vi "Test Real Matrix Type.vi"(9 "relative tolerance":dbl=-1.0, 10 "matrix type":T1=10 items=["Symmetric Positive Definite"=10, "Symmetric Positive Semi-Definite"=11, "Symmetric"=20, "Hermitian"=21], 11 "Input Matrix":T2) -> (0 "error":i32, 3 "is type?":bool)   [LabVIEW 2017, in "NI_AALPro.lvlib"]
doc: "Tests whether<B> Input Matrix</B> is a matrix of special type. Wire data to the <B>Input Matrix</B> input to determine the polymorphic instance to use or manually select the instance."
uses:
  NI_AALPro.lvlib
  RealMatrix.ctl
  Matrix Type for Test.ctl
  NI_Matrix.lvlib
panel:
  # "Test Matrix Type"
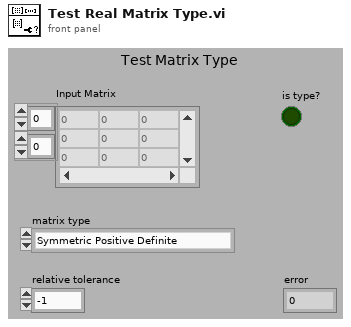
[diagram p1: front panel]
types:
  T1 = typedef "NI_AALPro.lvlib/Matrix Type for Test.ctl" = i32
  T2 = typedef "NI_Matrix.lvlib/RealMatrix.ctl" = dbl[][]
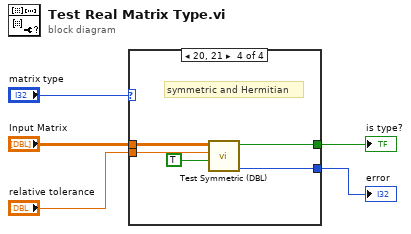
[diagram p0: block diagram]
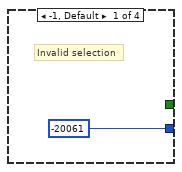
[diagram p2: hidden frame]
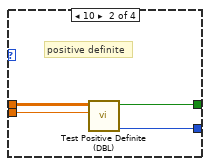
[diagram p3: hidden frame]
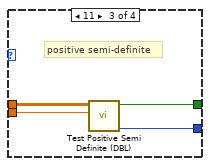
[diagram p4: hidden frame]
diagram:
  n1 = case shown="20, 21" "matrix type" {
    tunnel: "Input Matrix" -> [_ w10 w14 w19]
    tunnel: "relative tolerance" -> [_ w9 w13 w18]
    tunnel: [_ w7 w12 w17] -> w2
    tunnel: [-20061 ("return type") w8 w11 w16] -> w1
    frame -1, Default {
      # "Invalid selection"
    }
    frame 10 {
      # "positive definite"
      n2 = call "Test Positive Definite (DBL).vi"("relative tolerance"=w9, "Input Matrix"=w10) -> ("error"=w8:i32, "positive definite?"=w7:bool)  [unwired: 8 out]
    }
    frame 11 {
      # "positive semi-definite"
      n3 = call "Test Positive Semi Definite (DBL).vi"("relative tolerance"=w13, "Input Matrix"=w14) -> ("error"=w11:i32, "positive semidefinite?"=w12:bool)  [unwired: 8 out]
    }
    frame 20, 21 {
      # "symmetric and Hermitian"
      n4 = call "Test Symmetric (DBL).vi"("relative tolerance?"=TRUE, "tolerance"=w18, "Input Matrix"=w19) -> ("error"=w16:i32, "symmetric?"=w17:bool)  [unwired: 7 out]
    }
  }
  "error" <- w1
  "is type?" <- w2
